vi "CalInjGetState.vi"(8 "error in (no error)":errorcluster) -> (0 "error out":errorcluster, 3 "CalMotSta":T1)   [LabVIEW 2016]
uses:
  controls/MotorStates.ctl
  controls/RT-Variables.lvlib
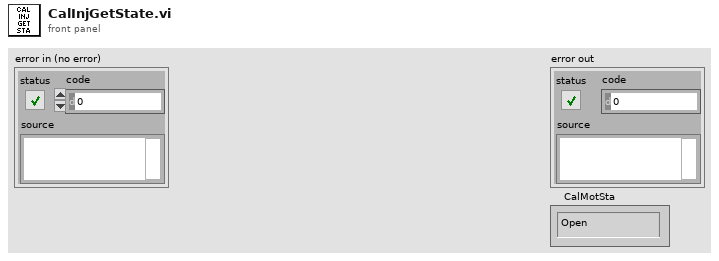
[diagram p1: front panel]
types:
  T1 = typedef "RT-Variables.lvlib/MotorStates.ctl" = enum16{"Open", "Close", "Moving", "Screwed"}
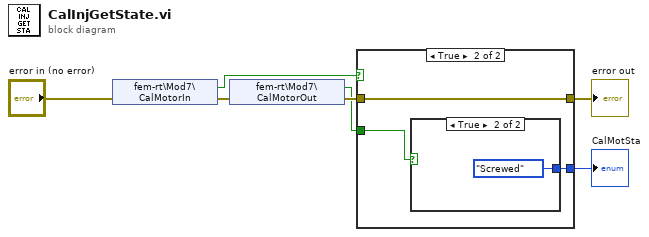
[diagram p0: block diagram]
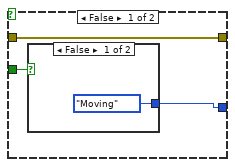
[diagram p2: hidden frame]
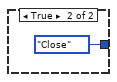
[diagram p3: hidden frame]
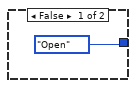
[diagram p4: hidden frame]
diagram:
  n1 = shared-variable "fem-rt\\Mod7\\CalMotorIn"(error in="error in (no error)") -> (w7:bool, error out=w3:errorcluster)
  n2 = shared-variable "fem-rt\\Mod7\\CalMotorOut"(error in=w3) -> (w1:bool, error out=w2:errorcluster)
  n3 = case shown="True" w7 {
    tunnel: w2 -> [w9 w15]
    tunnel: [w9 w15] -> w4
    tunnel: [w10 w14] -> w6
    tunnel: w1 -> [w8 w13]
    frame False {
      n4 = case shown="False" w8 {
        tunnel: [MotorStates."Moving" ("CalMotSta") MotorStates."Close" ("CalMotSta")] -> w10
        frame False {
        }
        frame True {
        }
      }
    }
    frame True {
      n5 = case shown="True" w13 {
        tunnel: [MotorStates."Open" ("CalMotSta") MotorStates."Screwed" ("CalMotSta")] -> w14
        frame False {
        }
        frame True {
        }
      }
    }
  }
  "error out" <- w4
  "CalMotSta" <- w6
